vi "Locate_in_Project.vi"   [LabVIEW 2009]
panel:
  # "Locate in Project\n\nHighlights a VI or other file in the project.\n\nPlease visit http://www.OpenG.org to learn about the\nOpen Source LabVIEW software movement.\n\nNOTICE -- YOU MUST LEAVE THIS NOTICE IN PLACE.  PER THE TERMS OF THE LICENSE BELOW, YOU MAY SUBLICENSE THIS SOFTWARE \nIN ANY WAY THAT DOES NOT CONFLICT WITH THIS LICENSE.\n\n### BSD License (http://www.opensource.org/licenses/bsd-license.php) Begin ###\n \nCopyright (c) 2007, Joe \"orko\" Sines <orko@wavecable.com>\nCopyright (c) 2007, Jim Kring <jim@jimkring.com>\nCopyright (c) 2011, Jonathon Green <jg@jgcode.net>\n\nAll rights reserved.\n\nRedistribution and use in source and binary forms, with or without modification, are permitted provided that the following conditions are met:\n\n    * Redistributions of source code must retain the above copyright notice, this list of conditions and the following disclaimer.\n    * Redistributions in binary form must reproduce the above copyright notice, this list of conditions and the following disclaimer in the \n       documentation and/or other materials provided with the distribution.\n    * Neither the name of SciWare, James Kring, Inc., nor the names of its contributors may be used to endorse or promote products derived \n       from this software without specific prior written permission.\n\nTHIS SOFTWARE IS PROVIDED BY THE COPYRIGHT HOLDERS AND CONTRIBUTORS \"AS IS\" AND ANY EXPRESS OR IMPLIED WARRANTIES, \nINCLUDING, BUT NOT LIMITED TO, THE IMPLIED WARRANTIES OF MERCHANTABILITY AND FITNESS FOR A PARTICULAR PURPOSE ARE \nDISCLAIMED. IN NO EVENT SHALL THE COPYRIGHT OWNER OR CONTRIBUTORS BE LIABLE FOR ANY DIRECT, INDIRECT, INCIDENTAL,\n SPECIAL, EXEMPLARY, OR CONSEQUENTIAL DAMAGES (INCLUDING, BUT NOT LIMITED TO, PROCUREMENT OF SUBSTITUTE GOODS OR \nSERVICES; LOSS OF USE, DATA, OR PROFITS; OR BUSINESS INTERRUPTION) HOWEVER CAUSED AND ON ANY THEORY OF LIABILITY, \nWHETHER IN CONTRACT, STRICT LIABILITY, OR TORT (INCLUDING NEGLIGENCE OR OTHERWISE) ARISING IN ANY WAY OUT OF THE USE \nOF THIS SOFTWARE, EVEN IF ADVISED OF THE POSSIBILITY OF SUCH DAMAGE.\n\n### BSD License End ###"
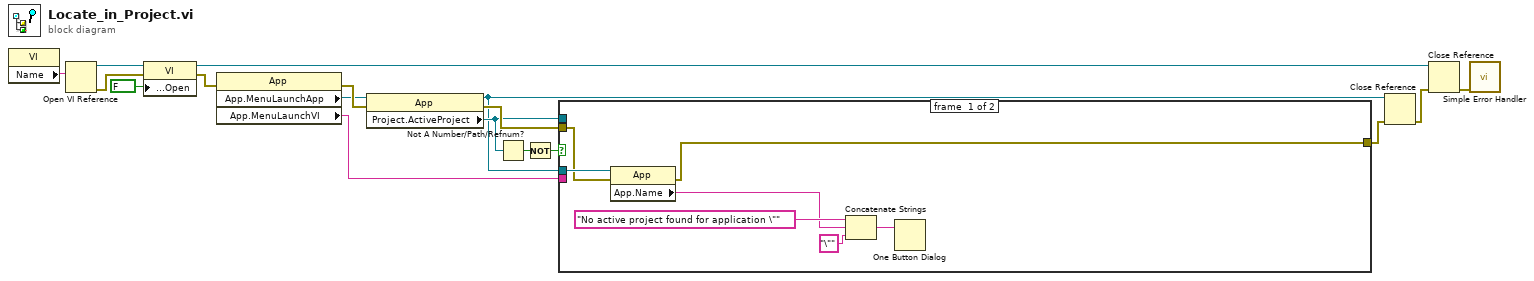
[diagram p0: block diagram]
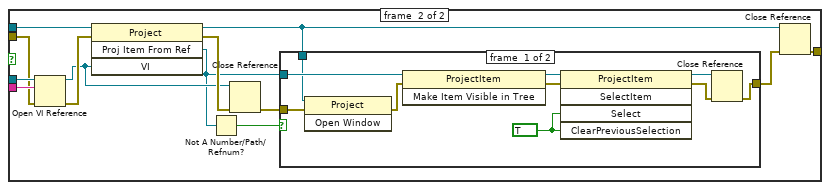
[diagram p2: hidden frame]
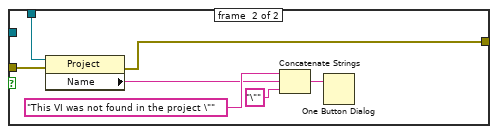
[diagram p3: hidden frame]
diagram:
  n1 = property class="VI"() -> ("Name"=w6:string)  [unwired: 2 in, 2 out]
  n2 = Open VI Reference(vi path=w6) -> (vi reference=w16:refnum<vi>, error out=w7:errorcluster)  [unwired: 5 in]
  n3 = property class="VI"(reference=w16, error in=w7, "Front Panel Window:Open"=FALSE) -> (reference out=w9:refnum<vi>, error out=w14:errorcluster)
  n4 = property class="App"(error in=w14) -> (error out=w8:errorcluster, "App.MenuLaunchApp"=w2:refnum<vi>, "App.MenuLaunchVI"=w15:string)  [unwired: 1 in, 1 out]
  n5 = property class="App"(reference=w2, error in=w8) -> (reference out=w1:refnum<vi>, error out=w13:errorcluster, "Project.ActiveProject"=w5:refnum<vi>)
  n6 = Not A Number/Path/Refnum?(number/path/refnum=w5) -> (NaN/Path/Refnum?=w4:bool)
  n7 = Not(x=w4) -> (.not. x?=w3:bool)
  n8 = case shown="True" w3 {
    tunnel: w15 -> [_ w35]
    tunnel: w13 -> [w20 w33]
    tunnel: [w19 w37] -> w12
    tunnel: w5 -> [_ w36]
    tunnel: w1 -> [w21 w34]
    frame #0 {
      n9 = property class="App"(reference=w21, error in=w20) -> (error out=w19:errorcluster, "App.Name"=w18:string)  [unwired: 1 out]
      n10 = Concatenate Strings("No active project found for application \"" ("message"), w18, "\"" ("string")) -> (w24:string)
      n11 = One Button Dialog(message=w24) -> ()  [unwired: 1 in, 1 out]
    }
    frame #1 {
      n12 = Open VI Reference(application reference (local)=w34, vi path=w35, error in (no error)=w33) -> (vi reference=w29:refnum<vi>, error out=w32:errorcluster)  [unwired: 3 in]
      n13 = invoke class="Project" method="Proj Item From Ref"(reference=w36, error in=w32, "VI"=w29) -> (reference out=w26:refnum<vi>, error out=w31:errorcluster, "ProjItemFromRef"=w27:refnum<vi>)  [unwired: 1 in, 1 out]
      n14 = Not A Number/Path/Refnum?(number/path/refnum=w27) -> (NaN/Path/Refnum?=w28:bool)
      n15 = Close Reference(reference=w29, error in (no error)=w31) -> (error out=w30:errorcluster)
      n16 = case shown="True" w28 {
        tunnel: [w38 w49] -> w25
        tunnel: w27 -> [w43 _]
        tunnel: w26 -> [w42 w54]
        tunnel: w30 -> [w41 w53]
        frame #0 {
          w46 = TRUE ("Select")
          n17 = invoke class="Project" method="Open Window"(reference=w42, error in=w41) -> (error out=w44:errorcluster)  [unwired: 1 in, 2 out]
          n18 = invoke class="ProjectItem" method="Make Item Visible in Tree"(reference=w43, error in=w44) -> (reference out=w47:refnum<vi>, error out=w45:errorcluster)  [unwired: 1 in, 1 out]
          n19 = invoke class="ProjectItem" method="SelectItem"(reference=w47, error in=w45, "Select"=w46, "ClearPreviousSelection"=w46) -> (reference out=w40:refnum<vi>, error out=w39:errorcluster)  [unwired: 1 in, 3 out]
          n20 = Close Reference(reference=w40, error in (no error)=w39) -> (error out=w38:errorcluster)
        }
        frame #1 {
          n21 = property class="Project"(reference=w54, error in=w53) -> (error out=w49:errorcluster, "Name"=w48:string)  [unwired: 1 out]
          n22 = Concatenate Strings("This VI was not found in the project \"" ("message"), w48, "\"" ("string")) -> (w52:string)
          n23 = One Button Dialog(message=w52) -> ()  [unwired: 1 in, 1 out]
        }
      }
      n24 = Close Reference(reference=w26, error in (no error)=w25) -> (error out=w37:errorcluster)
    }
  }
  n25 = Close Reference(reference=w1, error in (no error)=w12) -> (error out=w11:errorcluster)
  n26 = Close Reference(reference=w9, error in (no error)=w11) -> (error out=w10:errorcluster)
  n27 = call <vilib>:"Simple Error Handler.vi"("error in (no error)"=w10) -> ()  [unwired: 4 in, 5 out]
